vi "HEWH RLT Release Notifier References.vi"(8 "error in (no error)":errorcluster) -> (0 "error out":errorcluster)   [LabVIEW 2016]
uses:
  Type Definitions/HEWH Power Elements.ctl
  Utility/Type Definitions/UTILITY Notifier.ctl
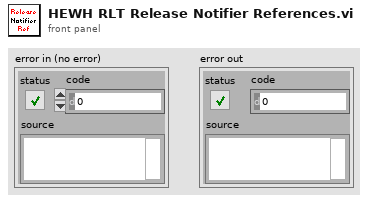
[diagram p1: front panel]
types:
  T1 = typedef "UTILITY Notifier.ctl" = enum16{"Set", "Read", "Release Ref"}
  T2 = typedef "HEWH Power Elements.ctl" = cluster{"UE":bool, "LE":bool, "COMP":bool, "FANS":bool}
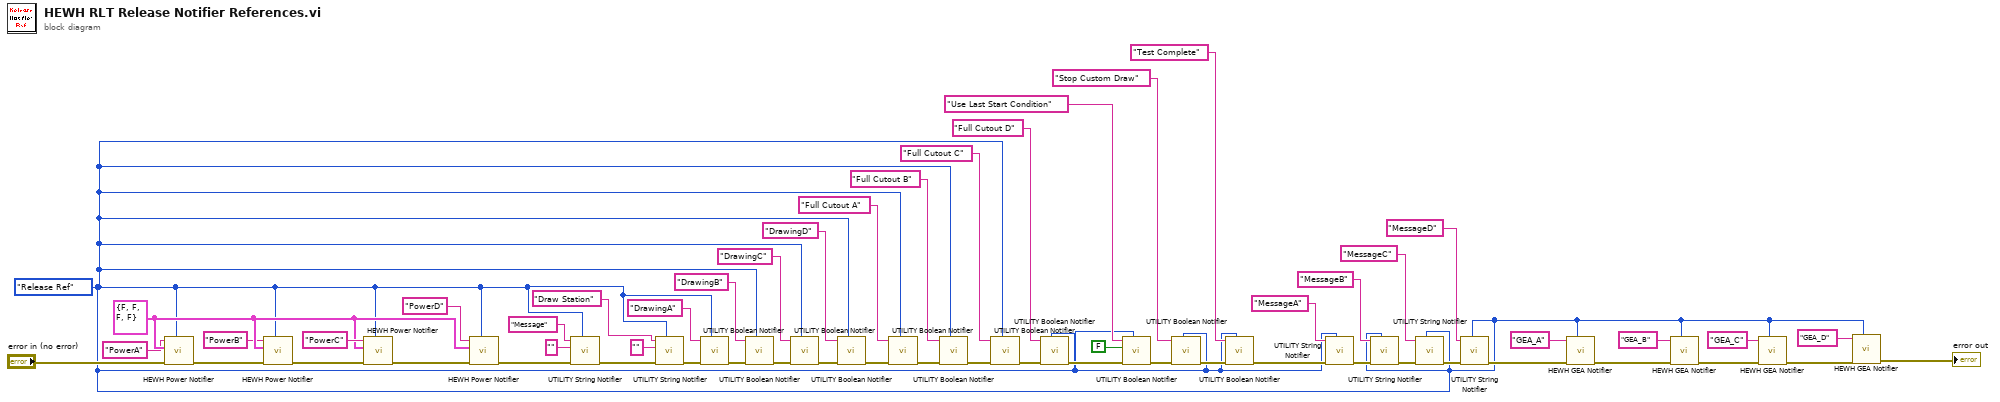
[diagram p0: block diagram]
diagram:
  w5 = UTILITY_Notifier."Release Ref" ("Status")
  w47 = T2 {"UE"=FALSE, "LE"=FALSE, "COMP"=FALSE, "FANS"=FALSE} ("Power Elements")
  n1 = call "HEWH Power Notifier.vi"("Status"=w5, "error in (no error)"="error in (no error)", "Set Status"=w47, "name (unnamed)"="PowerA") -> ("error out"=w42:errorcluster)  [unwired: 6 in, 1 out]
  n2 = call "HEWH Power Notifier.vi"("Status"=w5, "error in (no error)"=w42, "Set Status"=w47, "name (unnamed)"="PowerB") -> ("error out"=w44:errorcluster)  [unwired: 6 in, 1 out]
  n3 = call "HEWH Power Notifier.vi"("Status"=w5, "error in (no error)"=w44, "Set Status"=w47, "name (unnamed)"="PowerC") -> ("error out"=w45:errorcluster)  [unwired: 6 in, 1 out]
  n4 = call "HEWH Power Notifier.vi"("Status"=w5, "error in (no error)"=w45, "Set Status"=w47, "name (unnamed)"="PowerD") -> ("error out"=w52:errorcluster)  [unwired: 6 in, 1 out]
  n5 = call "UTILITY String Notifier.vi"("Status"=w5, "error in (no error)"=w52, "Set Status"="", "name (unnamed)"="Message") -> ("error out"=w54:errorcluster)  [unwired: 6 in, 1 out]
  n6 = call "UTILITY String Notifier.vi"("Status"=w5, "error in (no error)"=w54, "Set Status"="", "name (unnamed)"="Draw Station") -> ("error out"=w36:errorcluster)  [unwired: 6 in, 1 out]
  n7 = call "UTILITY Boolean Notifier.vi"("Status"=w5, "error in (no error)"=w36, "name (unnamed)"="DrawingA") -> ("error out"=w35:errorcluster)  [unwired: 7 in, 1 out]
  n8 = call "UTILITY Boolean Notifier.vi"("Status"=w5, "error in (no error)"=w35, "name (unnamed)"="DrawingB") -> ("error out"=w34:errorcluster)  [unwired: 7 in, 1 out]
  n9 = call "UTILITY Boolean Notifier.vi"("Status"=w5, "error in (no error)"=w34, "name (unnamed)"="DrawingC") -> ("error out"=w33:errorcluster)  [unwired: 7 in, 1 out]
  n10 = call "UTILITY Boolean Notifier.vi"("Status"=w5, "error in (no error)"=w33, "name (unnamed)"="DrawingD") -> ("error out"=w28:errorcluster)  [unwired: 7 in, 1 out]
  n11 = call "UTILITY Boolean Notifier.vi"("Status"=w5, "error in (no error)"=w28, "name (unnamed)"="Full Cutout A") -> ("error out"=w27:errorcluster)  [unwired: 7 in, 1 out]
  n12 = call "UTILITY Boolean Notifier.vi"("Status"=w5, "error in (no error)"=w27, "name (unnamed)"="Full Cutout B") -> ("error out"=w26:errorcluster)  [unwired: 7 in, 1 out]
  n13 = call "UTILITY Boolean Notifier.vi"("Status"=w5, "error in (no error)"=w26, "name (unnamed)"="Full Cutout C") -> ("error out"=w25:errorcluster)  [unwired: 7 in, 1 out]
  n14 = call "UTILITY Boolean Notifier.vi"("Status"=w5, "error in (no error)"=w25, "name (unnamed)"="Full Cutout D") -> ("error out"=w22:errorcluster)  [unwired: 7 in, 1 out]
  n15 = call "UTILITY Boolean Notifier.vi"("Status"=w5, "error in (no error)"=w22, "Set Status"=FALSE, "name (unnamed)"="Use Last Start Condition") -> ("error out"=w21:errorcluster)  [unwired: 6 in, 1 out]
  n16 = call "UTILITY Boolean Notifier.vi"("Status"=w5, "error in (no error)"=w21, "name (unnamed)"="Stop Custom Draw") -> ("error out"=w20:errorcluster)  [unwired: 7 in, 1 out]
  n17 = call "UTILITY Boolean Notifier.vi"("Status"=w5, "error in (no error)"=w20, "name (unnamed)"="Test Complete") -> ("error out"=w17:errorcluster)  [unwired: 7 in, 1 out]
  n18 = call "UTILITY String Notifier.vi"("Status"=w5, "error in (no error)"=w17, "name (unnamed)"="MessageA") -> ("error out"=w14:errorcluster)  [unwired: 7 in, 1 out]
  n19 = call "UTILITY String Notifier.vi"("Status"=w5, "error in (no error)"=w14, "name (unnamed)"="MessageB") -> ("error out"=w15:errorcluster)  [unwired: 7 in, 1 out]
  n20 = call "UTILITY String Notifier.vi"("Status"=w5, "error in (no error)"=w15, "name (unnamed)"="MessageC") -> ("error out"=w16:errorcluster)  [unwired: 7 in, 1 out]
  n21 = call "UTILITY String Notifier.vi"("Status"=w5, "error in (no error)"=w16, "name (unnamed)"="MessageD") -> ("error out"=w10:errorcluster)  [unwired: 7 in, 1 out]
  n22 = call "HEWH GEA Notifier.vi"("Status"=w5, "error in (no error)"=w10, "name (unnamed)"="GEA_A") -> ("error out"=w9:errorcluster)  [unwired: 7 in, 1 out]
  n23 = call "HEWH GEA Notifier.vi"("Status"=w5, "error in (no error)"=w9, "name (unnamed)"="GEA_B") -> ("error out"=w8:errorcluster)  [unwired: 7 in, 1 out]
  n24 = call "HEWH GEA Notifier.vi"("Status"=w5, "error in (no error)"=w8, "name (unnamed)"="GEA_C") -> ("error out"=w7:errorcluster)  [unwired: 7 in, 1 out]
  n25 = call "HEWH GEA Notifier.vi"("Status"=w5, "error in (no error)"=w7, "name (unnamed)"="GEA_D") -> ("error out"=→"error out":errorcluster)  [unwired: 7 in, 1 out]
